vi "MyFPGA DIO_Encoder.vi"(0 "DIO.1:0.OUT":fxp<+,2,2> format="%02b", 1 "DIO.1:0.DIR":fxp<+,2,2> format="%02b", 5 "QE.CNFG":u8, 6 "DIO.1/QE.B":refnum<k21>, 7 "SELECT":bool, 8 "DIO.0/QE.A":refnum<k21>) -> (14 "DIO.1:0.IN":fxp<+,2,2> format="%02b", 18 "QE.CNTR":u32, 19 "QE.STAT":u8 format="%08b")   [LabVIEW 2019]
doc: "This VI switches between the DIO functionality and the Encoder functionality for the specified FPGA I/O channels.\n- If <b>SELECT</b> is FALSE, DIO0 and DIO1 are enabled.\n- If <b>SELECT</b> is TRUE, Encoder Phase A and Phase B are enabled."
panel:
  # "This VI switches between the DIO functionality and the Encoder functionality for the specified FPGA I/O channels.\n- If SELECT is FALSE, DIO0 and DIO1 are enabled.\n- If SELECT is TRUE, Encoder Phase A and Phase B are enabled."
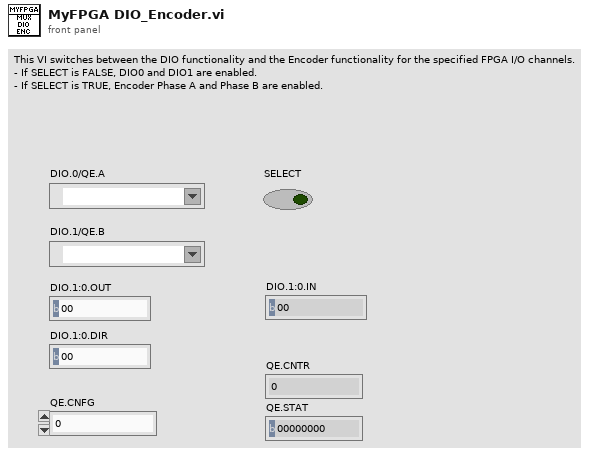
[diagram p1: front panel]
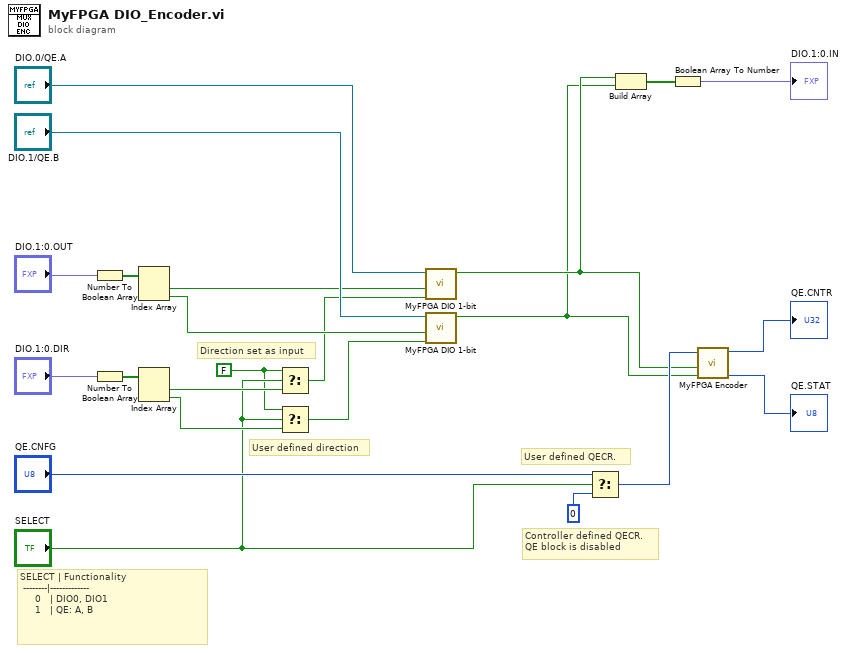
[diagram p0: block diagram]
diagram:
  w3 = FALSE ("t")
  # "User defined direction"
  # "Direction set as input"
  # "SELECT | Functionality \n --------|-------------\n     0   | DIO0, DIO1\n     1   | QE: A, B"
  # "Controller defined QECR.\nQE block is disabled"
  # "User defined QECR."
  n1 = Number To Boolean Array(number="DIO.1:0.OUT") -> (Boolean array=w14:bool[])
  n2 = Number To Boolean Array(number="DIO.1:0.DIR") -> (Boolean array=w13:bool[])
  n3 = Index Array(array=w14) -> (element #1=w10:bool, element #2=w9:bool)  [unwired: 2 in]
  n4 = Index Array(array=w13) -> (element #1=w8:bool, element #2=w7:bool)  [unwired: 2 in]
  n5 = Select(t=w3, s="SELECT", f=w8) -> (s? t:f=w5:bool)
  n6 = Select(t=w3, s="SELECT", f=w7) -> (s? t:f=w4:bool)
  n7 = call "MyFPGA DIO 1-bit.vi"("DIR"=w5, "OUT"=w10, "DIO Refnum"="DIO.0/QE.A") -> ("IN"=w2:bool)  [unwired: 8 in]
  n8 = call "MyFPGA DIO 1-bit.vi"("DIR"=w4, "OUT"=w9, "DIO Refnum"="DIO.1/QE.B") -> ("IN"=w1:bool)  [unwired: 8 in]
  n9 = Select(t="QE.CNFG", s="SELECT", f=u8 0) -> (s? t:f=w20:u8)
  n10 = Build Array(w2, w1) -> (w12:bool[])
  n11 = Boolean Array To Number(Boolean array=w12) -> (number=→"DIO.1:0.IN":fxp<+,2,2>)
  n12 = call "MyFPGA Encoder.vi"("Phase B"=w1, "Phase A"=w2, "CNFG"=w20) -> ("STAT"=→"QE.STAT":u8, "CNTR"=→"QE.CNTR":u32)  [unwired: 7 in]
